vi "Junk.vi"() -> ()   [LabVIEW 2016]
uses:
  <vilib>/rvi/Emulation/niFpgaGetClockAttributes.vi
  <vilib>/rvi/Emulation/niFpgaSctlEmulationGetInTimedLoop.vi
  <vilib>/rvi/Emulation/niFpgaEmulationReportErrorSimple.vi
  <vilib>/rvi/eio/common/nirviEmuTemplateMethod_errors.vi
  <vilib>/rvi/Emulation/niFpgaCriticalErrorInLSC.vi
  <vilib>/eio/EIOMethodNode/EIOMethodNode.xnode
panel:
  out "Numeric":i32
  out "Data 2":u8
  out "Data":u8
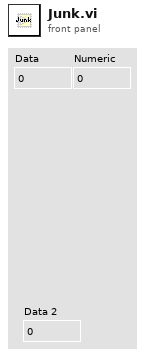
[diagram p1: front panel]
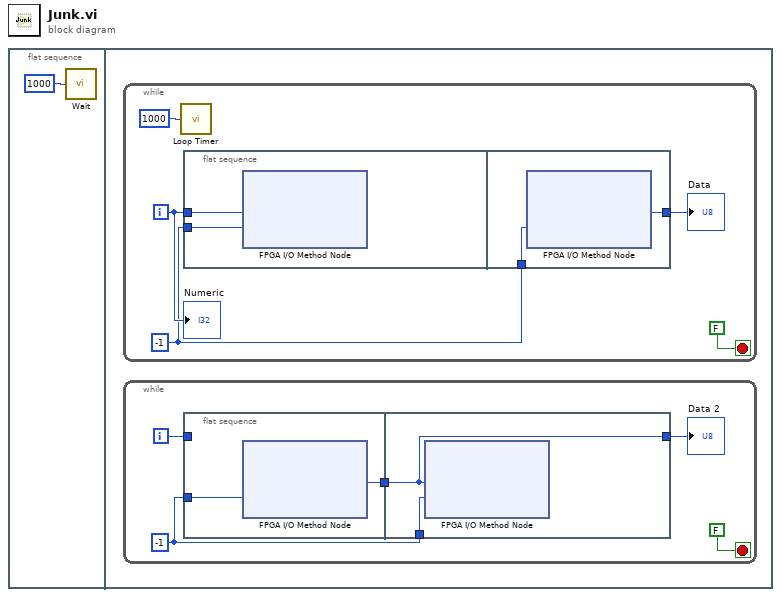
[diagram p0: block diagram]
diagram:
  n1 = flat-sequence {
    frame #0 {
      n2 = call "Wait"("Count(mSec)"=u32 1000) -> ()  [unwired: 1 out]
    }
    frame #1 {
      n3 = while {
        i -> [w15]
        stop <- FALSE stop-if-true
        w11 = -1 ("Timeout (ms)")
        n4 = call "Loop Timer"("Count(mSec)"=u32 1000) -> ()  [unwired: 1 out]
        n5 = flat-sequence {
          tunnel: w15 -> [w17]
          tunnel: w11 -> [w16]
          tunnel: [w19] -> w12
          tunnel: w11 -> [w18]
          frame #0 {
            n6 = xnode "FPGA I/O Method Node"("Data"=w17, "Timeout (ms)"=w16) -> ()  [unwired: 1 in, 2 out]
          }
          frame #1 {
            n7 = xnode "FPGA I/O Method Node"("Timeout (ms)"=w18) -> ("Data"=w19:u8)  [unwired: 1 in, 2 out]
          }
        }
        "Data" <- w12
        "Numeric" <- w15
      }
      n8 = while {
        i -> [w6]
        stop <- FALSE stop-if-true
        w3 = -1 ("Timeout (ms)")
        n9 = flat-sequence {
          tunnel: w6 -> [_]
          tunnel: w3 -> [w8]
          tunnel: [w7] -> w2
          tunnel: [w9] -> w4
          tunnel: w3 -> [w10]
          tunnel: w2 -> [w9]
          frame #0 {
            n10 = xnode "FPGA I/O Method Node"("Timeout (ms)"=w8) -> ("Data"=w7:u8)  [unwired: 1 in, 2 out]
          }
          frame #1 {
            n11 = xnode "FPGA I/O Method Node"("Data"=w9, "Timeout (ms)"=w10) -> ()  [unwired: 1 in, 2 out]
          }
        }
        "Data 2" <- w4
      }
    }
  }
